vi "Gripper Status.vi"(8 "error in (no error)":errorcluster, 11 "Robotiq in":refnum<class "Robotiq.lvclass">) -> (0 "error out":errorcluster, 2 "Gripper Status":T1, 3 "Robotiq out":refnum<class "Robotiq.lvclass">)   [LabVIEW 2013, in "Robotiq.lvclass"]
uses:
  Robotiq.lvclass
  Controls/Gripper Status.ctl
  Controls/Finger Status.ctl
  Robotiq.lvclass/Robotiq.ctl
  <vilib>/NI Modbus.llb/MB Ethernet Master Query Read Input Registers (poly).vi
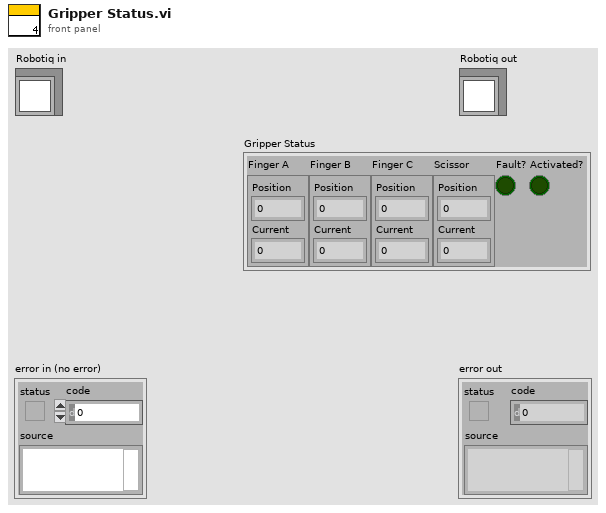
[diagram p1: front panel]
types:
  T1 = typedef "Gripper Status.ctl" = cluster{"Finger A":T2, "Finger B":T2, "Finger C":T2, "Scissor":T2, "Fault?":bool, "Activated?":bool}
  T2 = typedef "Finger Status.ctl" = cluster{"Position":dbl, "Current":dbl}
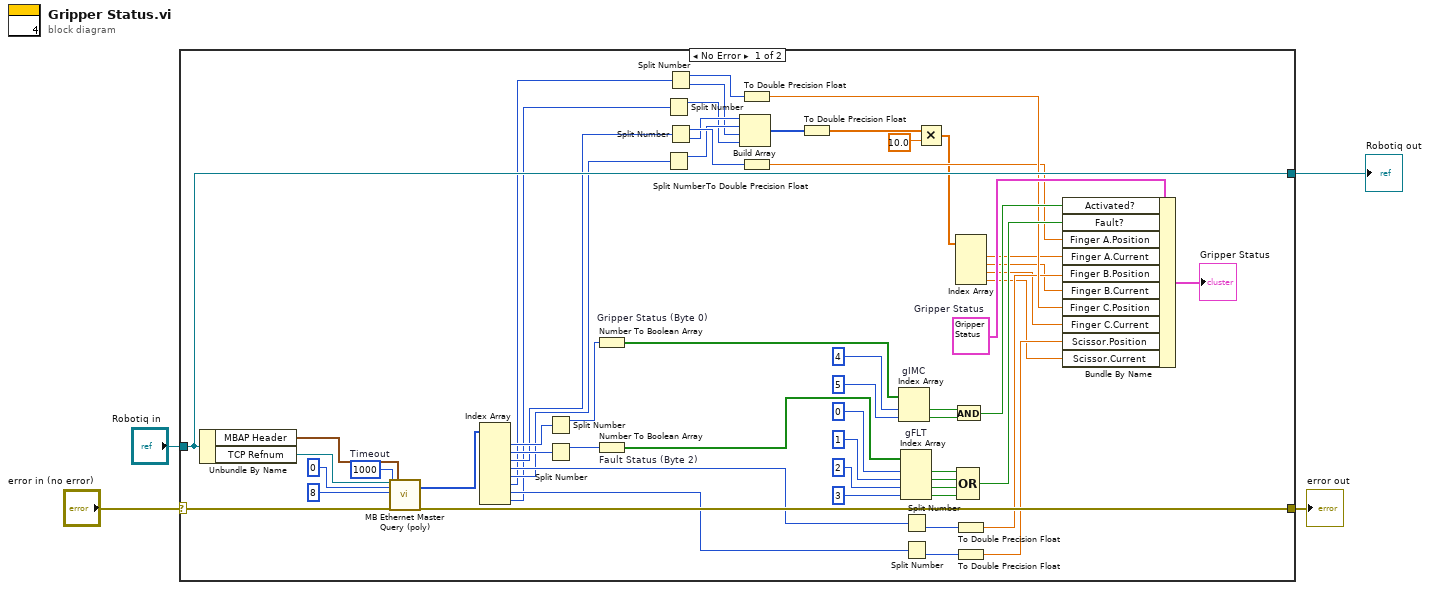
[diagram p0: block diagram]
diagram:
  n1 = case shown="No Error" "error in (no error)" {
    selector: "error in (no error)" -> [w57 w63]
    tunnel: [w56 w63] -> w3
    tunnel: [w61 w62] -> w1
    tunnel: "Robotiq in" -> [w61 w62]
    frame No Error {
      w5 = 1000  # Timeout
      w53 = T1 {"Finger A"={"Position"=0.0, "Current"=0.0}, "Finger B"={"Position"=0.0, "Current"=0.0}, "Finger C"={"Position"=0.0, "Current"=0.0}, "Scissor"={"Position"=0.0, "Current"=0.0}, "Fault?"=FALSE, "Activated?"=FALSE}  # Gripper Status
      n2 = Unbundle By Name(w61) -> ("MBAP Header"=w60:cluster{"Transaction ID":u16, "Unit ID":u8}, "TCP Refnum"=w59:refnum<k5>)
      n3 = call-poly <vilib>:"MB Ethernet Master Query (poly).vi"("TCP Connection Refnum in"=w59, "Starting Address"=u16 0 ("Address"), "Quantity"=u16 8, "Timeout"=w5, "error in"=w57, "MBAP Header"=w60) -> ("Input Registers"=w54:u16[], "error out"=w56:errorcluster)  [unwired: 10 in, 2 out]
      n4 = Index Array(array=w54) -> (element #1=w51:u16, element #2=w43:u16, element #3=w31:u16, element #4=w30:u16, element #5=w29:u16, element #6=w28:u16, element #7=w27:u16, element #8=w26:u16)  [unwired: 8 in]
      n5 = Split Number(x=w51) -> (hi(x)=w50:u8)  [unwired: 1 out]
      n6 = Split Number(x=w43) -> (hi(x)=w42:u8)  [unwired: 1 out]
      n7 = Number To Boolean Array "Gripper Status (Byte 0)"(number=w50) -> (Boolean array=w49:bool[])
      n8 = Number To Boolean Array "Fault Status (Byte 2)"(number=w42) -> (Boolean array=w41:bool[])
      n9 = Split Number(x=w26) -> (hi(x)=w14:u8)  [unwired: 1 out]
      n10 = Split Number(x=w29) -> (hi(x)=w16:u8)  [unwired: 1 out]
      n11 = Split Number(x=w28) -> (hi(x)=w23:u8, lo(x)=w15:u8)
      n12 = Split Number(x=w31) -> (hi(x)=w19:u8, lo(x)=w17:u8)
      n13 = Build Array(w17, w16, w15, w14) -> (w13:u8[])
      n14 = To Double Precision Float(number=w23) -> (double precision float=w22:dbl)
      n15 = To Double Precision Float(number=w19) -> (double precision float=w18:dbl)
      n16 = To Double Precision Float(number=w13) -> (double precision float=w12:dbl[])
      n17 = Index Array "gIMC"(array=w49, index #1=4 ("index"), index #2=5 ("index")) -> (element #1=w45:bool, element #2=w46:bool)
      n18 = Index Array "gFLT"(array=w41, index #1=0 ("index"), index #2=1 ("index"), index #3=2 ("index"), index #4=3 ("index")) -> (element #1=w36:bool, element #2=w35:bool, element #3=w34:bool, element #4=w33:bool)
      n19 = Split Number(x=w30) -> (lo(x)=w21:u8)  [unwired: 1 out]
      n20 = Split Number(x=w27) -> (lo(x)=w24:u8)  [unwired: 1 out]
      n21 = Multiply(x=w12, y=10.0) -> (x*y=w10:dbl[])
      n22 = And(x=w45, y=w46) -> (x .and. y?=w44:bool)
      n23 = Index Array(array=w10) -> (element #1=w9:dbl, element #2=w8:dbl, element #3=w7:dbl, element #4=w6:dbl)  [unwired: 4 in]
      n24 = To Double Precision Float(number=w21) -> (double precision float=w20:dbl)
      n25 = To Double Precision Float(number=w24) -> (double precision float=w25:dbl)
      n26 = Compound Arithmetic op=OR(w36, w35, w34, w33) -> (w32:bool)
      n27 = Bundle By Name(cluster=w53, "Activated?"=w44, "Fault?"=w32, "Finger A.Position"=w18, "Finger A.Current"=w9, "Finger B.Position"=w20, "Finger B.Current"=w8, "Finger C.Position"=w22, "Finger C.Current"=w7, "Scissor.Position"=w25, "Scissor.Current"=w6) -> (→"Gripper Status":T1)
    }
    frame Error {
    }
  }
  "error out" <- w3
  "Robotiq out" <- w1
